vi "Rd Wr Filter Wheel Settings obsolete.vi"(8 "error in (no error)":errorcluster, 9 "Name":string, 10 "Write? (F:Read)":bool, 11 "Filter Wheel Info":T3) -> (0 "error out":errorcluster, 3 "Filter Wheel Info":T2={"Num Wheels"=4, "Filters"=[{"Names"=["Grism", "blocked", "open", "VPH", "J", "Y"], "Relative Position"=[100, 1000, 2000, 3000, 4000, 5000], "Wheel Name"="FW YJ"}, {"Names"=["Grism", "blocked", "open", "VPH", "H", "K"], "Relative Position"=[10000, 7000, 8000, 8000, 7000, 10000], "Wheel Name"="FW HK"}, {"Names"=["135", "blocked", "80", "open 1", "250", "open"], "Relative Position"=[6000, 6000, 7000, 7000, 7000, 7000], "Wheel Name"="Slit wheel"}, {"Names"=["A", "B", "C", "D", "E", "F", "G", "H"], "Relative Position"=[5000, 5000, 5000, 5000, 5000, 5000, 5000, 5000], "Wheel Name"="FW aux"}], "Invalid Combinations"=[], "Addr"="", "Name"="PRIME", "Simulate"=FALSE})   [LabVIEW 2019]
uses:
  Filter Wheel Object/Filter Wheel Details.ctl
  Filter Wheel Object/Filter Wheel.lvclass
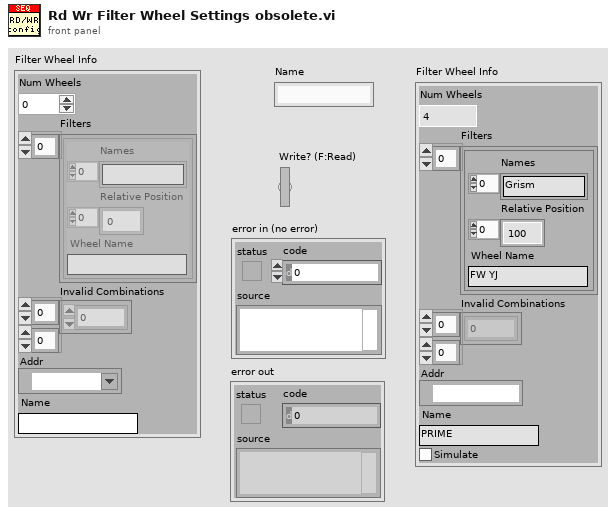
[diagram p1: front panel]
types:
  T1 = typedef "Filter Wheel.lvclass/Filter Wheel Details.ctl" = cluster{"Names":string[], "Relative Position":i32[], "Wheel Name":string}
  T2 = cluster{"Num Wheels":i32, "Filters":T1[], "Invalid Combinations":i32[][], "Addr":refnum<visa-resource-name>, "Name":string, "Simulate":bool}
  T3 = cluster{"Num Wheels":i32, "Filters":T1[], "Invalid Combinations":i32[][], "Addr":refnum<visa-resource-name>, "Name":string}
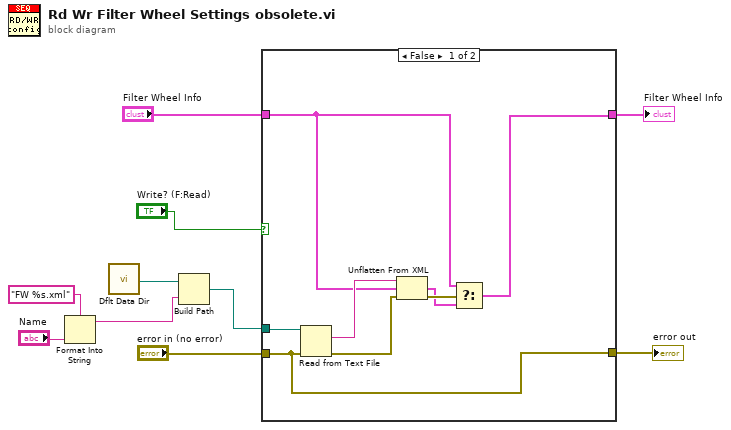
[diagram p0: block diagram]
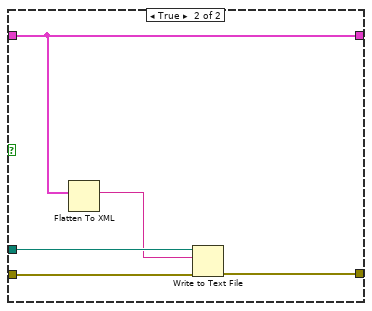
[diagram p2: hidden frame]
diagram:
  n1 = Format Into String(format string="FW %s.xml", "Name") -> (resulting string=w1:string)  [unwired: 2 in, 1 out]
  n2 = call <vilib>:"Dflt Data Dir.vi"() -> ("App:Default Data Directory"=w7:path)
  n3 = Build Path(base path=w7, name or relative path=w1) -> (appended path=w6:path)
  n4 = case shown="False" "Write? (F:Read)" {
    tunnel: "error in (no error)" -> [w11 w23]
    tunnel: "Filter Wheel Info" -> [w14 w19]
    tunnel: w6 -> [w18 w22]
    tunnel: [w11 w20] -> w5
    tunnel: [w12 w19] -> w4
    frame False {
      n5 = Read from Text File(file (use dialog)=w18, error in=w11) -> (text=w17:string, error out=w16:errorcluster)  [unwired: 2 in, 2 out]
      n6 = Unflatten From XML(xml string=w17, type=w14, error in (no error)=w16) -> (value=w13:T3, error out=w15:errorcluster)
      n7 = Select(t=w14, s=w15, f=w13) -> (s? t:f=w12:T3)
    }
    frame True {
      n8 = Flatten To XML(anything=w19) -> (xml string=w21:string)
      n9 = Write to Text File(file (use dialog)=w22, text=w21, error in=w23) -> (error out=w20:errorcluster)  [unwired: 1 in, 2 out]
    }
  }
  "error out" <- w5
  "Filter Wheel Info" <- w4
